vi "Match tags bold underline italic strikeout.vi"(11 "Text":string="Il <b>é<b>tait</b> une fois un jongleur qui ne savait pas<i> jongler alors il utilisa un </u>arc.") -> (1 "Array":T3(array[cluster])=[{"Text type"=enum."Text", "Text"="Il <b>é<b>tait</b> une fois un jongleur qui ne savait pas<i> jongler alors il utilisa un </u>arc.", "Hyperlink"=""}, {"Text type"=enum."empty", "Text"="", "Hyperlink"=""}, {"Text type"=enum."empty", "Text"="", "Hyperlink"=""}], 3 "Find tag ?":bool)   [LabVIEW 2019, in "Exaprom PDF.lvlib"]
doc: "Version 1.0\nDeveloped by Jean-Marc Simard\nCopyright © 2010, Exaprom Inc.\nAll rights reserved.\nLicense: BSD"
uses:
  Controls/Text Controls/Text type.ctl
  Exaprom PDF.lvlib
panel:
  out "Array 3":T1(array[cluster])=[{"Text"="</b>", "offset past match"=14}, {"Text"="</u>", "offset past match"=89}]
  out "Array 2":T1(array[cluster])=[{"Text"="<b>", "offset past match"=3}, {"Text"="<b>", "offset past match"=7}, {"Text"="<i>", "offset past match"=57}]
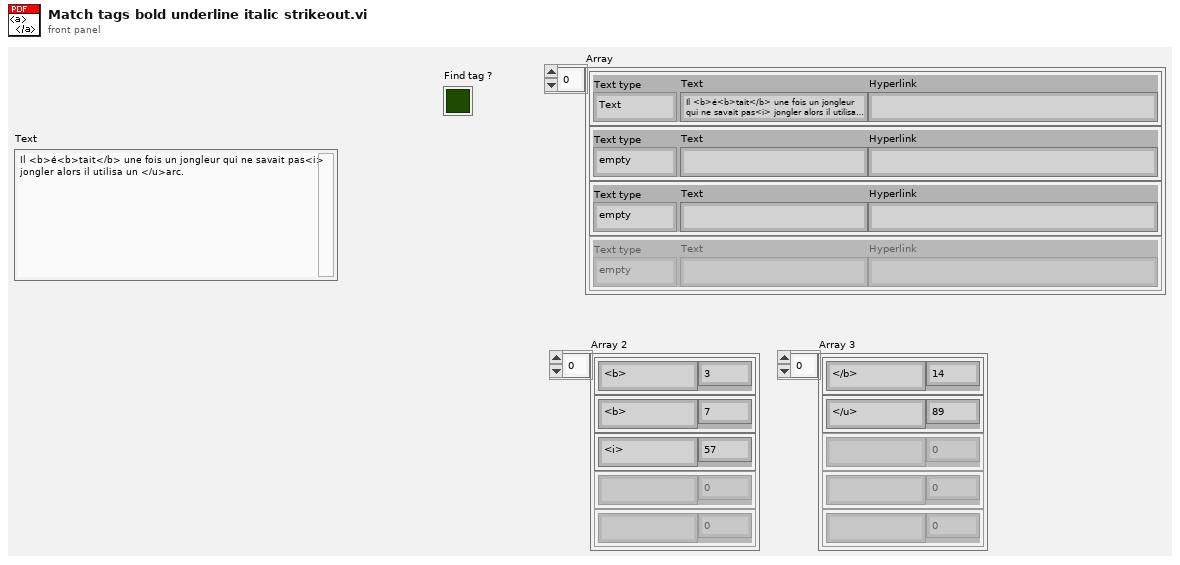
[diagram p1: front panel]
types:
  T1 = cluster{"Text":string, "offset past match":i32}[]
  T2 = typedef "Exaprom PDF.lvlib/Text type.ctl" = enum16{"empty", "Text", "Hyperlink"}
  T3 = cluster{"Text type":T2, "Text":string, "Hyperlink":string}[]
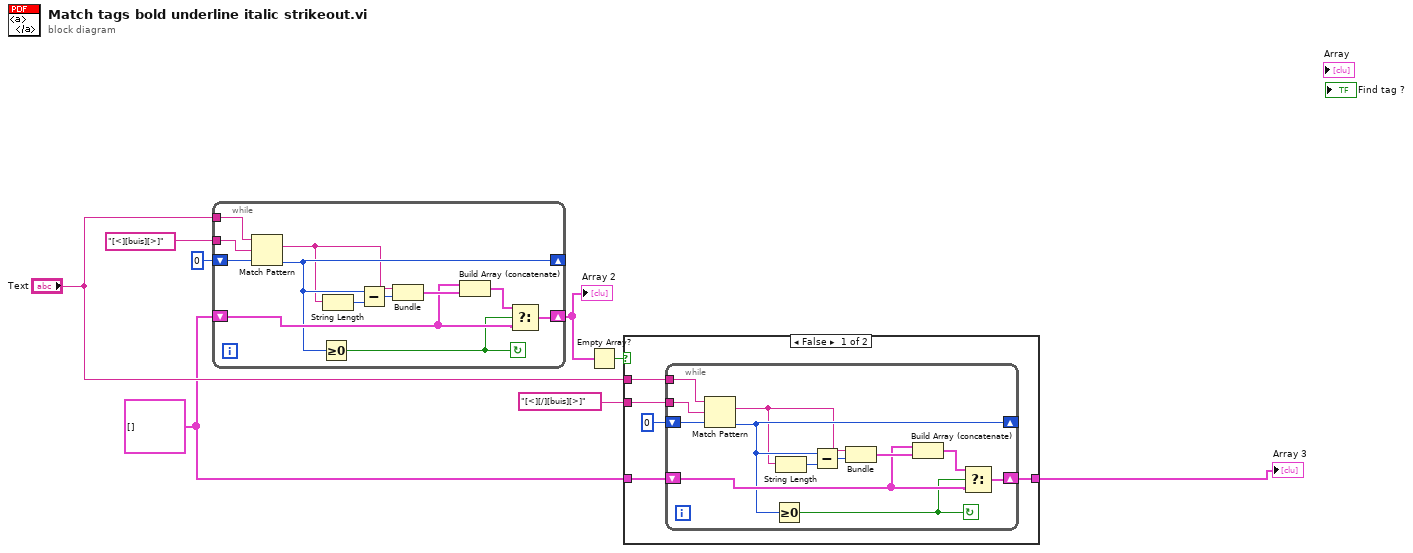
[diagram p0: block diagram]
diagram:
  w1 = T1 []
  n1 = while {
    tunnel: "[<][buis][>]" -> [w20]
    shift-right: [w19] -> w5
    shift-left: w1 -> [w16]
    shift-right: [w12] -> _
    shift-left: 0 -> [w15]
    tunnel: "Text" -> [w13]
    stop <- w14 continue-if-true
    n2 = Match Pattern(string=w13, regular expression=w20, offset (0)=w15) -> (match substring=w11:string, offset past match=w12:i32)  [unwired: 2 out]
    n3 = Greater Or Equal To 0?(x=w12) -> (x >= 0?=w14:bool)
    n4 = String Length(string=w11) -> (length=w10:i32)
    n5 = Subtract(x=w12, y=w10) -> (x-y=w9:i32)
    n6 = Bundle("Text"=w11, w9) -> (w18:cluster{"Text":string, i32})  [unwired: 1 out]
    n7 = Build Array (concatenate)(w16, w18) -> (w17:T1)
    n8 = Select(t=w17, s=w14, f=w16) -> (s? t:f=w19:T1)
  }
  "Array 2" <- w5
  n9 = Empty Array?(array=w5) -> (empty?=w8:bool)
  n10 = case shown="False" w8 {
    tunnel: "Text" -> [w24 _]
    tunnel: w1 -> [w23 w38]
    tunnel: "[<][/][buis][>]" -> [w22 _]
    tunnel: [w21 w38] -> w6
    frame False {
      n11 = while {
        tunnel: w22 -> [w37]
        shift-right: [w36] -> w21
        shift-left: w23 -> [w33]
        shift-right: [w29] -> _
        shift-left: 0 -> [w32]
        tunnel: w24 -> [w30]
        stop <- w31 continue-if-true
        n12 = Match Pattern(string=w30, regular expression=w37, offset (0)=w32) -> (match substring=w28:string, offset past match=w29:i32)  [unwired: 2 out]
        n13 = Greater Or Equal To 0?(x=w29) -> (x >= 0?=w31:bool)
        n14 = String Length(string=w28) -> (length=w27:i32)
        n15 = Subtract(x=w29, y=w27) -> (x-y=w26:i32)
        n16 = Bundle("Text"=w28, w26) -> (w35:cluster{"Text":string, i32})  [unwired: 1 out]
        n17 = Build Array (concatenate)(w33, w35) -> (w34:T1)
        n18 = Select(t=w34, s=w31, f=w33) -> (s? t:f=w36:T1)
      }
    }
    frame True {
    }
  }
  "Array 3" <- w6
